vi "FilterAndReorderChannels.vi"(8 "error in (no error)":errorcluster, 10 "channels":T9[](array[typedef]), 11 "device":T1) -> (0 "error out":errorcluster, 2 "acquisition channels (in acquisition order)":T9[](array[typedef]))   [LabVIEW 2017, in "CmsAcquisition.lvlib"]
uses:
  <vilib>/addons/InsightCM/Devices/Shared/Cms/CmsAcquisition/CmsAcquisition.lvlib
  <vilib>/addons/InsightCM/MessageBus/Base/controls/R2_Channel.ctl
  <vilib>/addons/InsightCM/MessageBus/Base/controls/KeyValuePair.ctl
  <vilib>/addons/InsightCM/MessageBus/Base/controls/Metric.ctl
  <vilib>/addons/InsightCM/MessageBus/Base/controls/R2_Device.ctl
  <vilib>/addons/InsightCM/MessageBus/Base/controls/DeviceState.ctl
  <vilib>/addons/InsightCM/MessageBus/Base/controls/R2_DataGroup.ctl
  <vilib>/addons/InsightCM/MessageBus/Base/controls/OperatingState.ctl
  <vilib>/addons/InsightCM/MessageBus/Base/controls/Trigger.ctl
  <vilib>/addons/InsightCM/MessageBus/Base/controls/Condition.ctl
  <vilib>/addons/InsightCM/MessageBus/Base/controls/BurstModeTrigger.ctl
  <vilib>/addons/InsightCM/Utilities/PropertyHelpers/PropertyHelpers.lvlib
panel:
  out "hardware channel name (in acquisition order)":string[](array[string])
  out "channel IDs (in acquisition order)":string[](array[string])
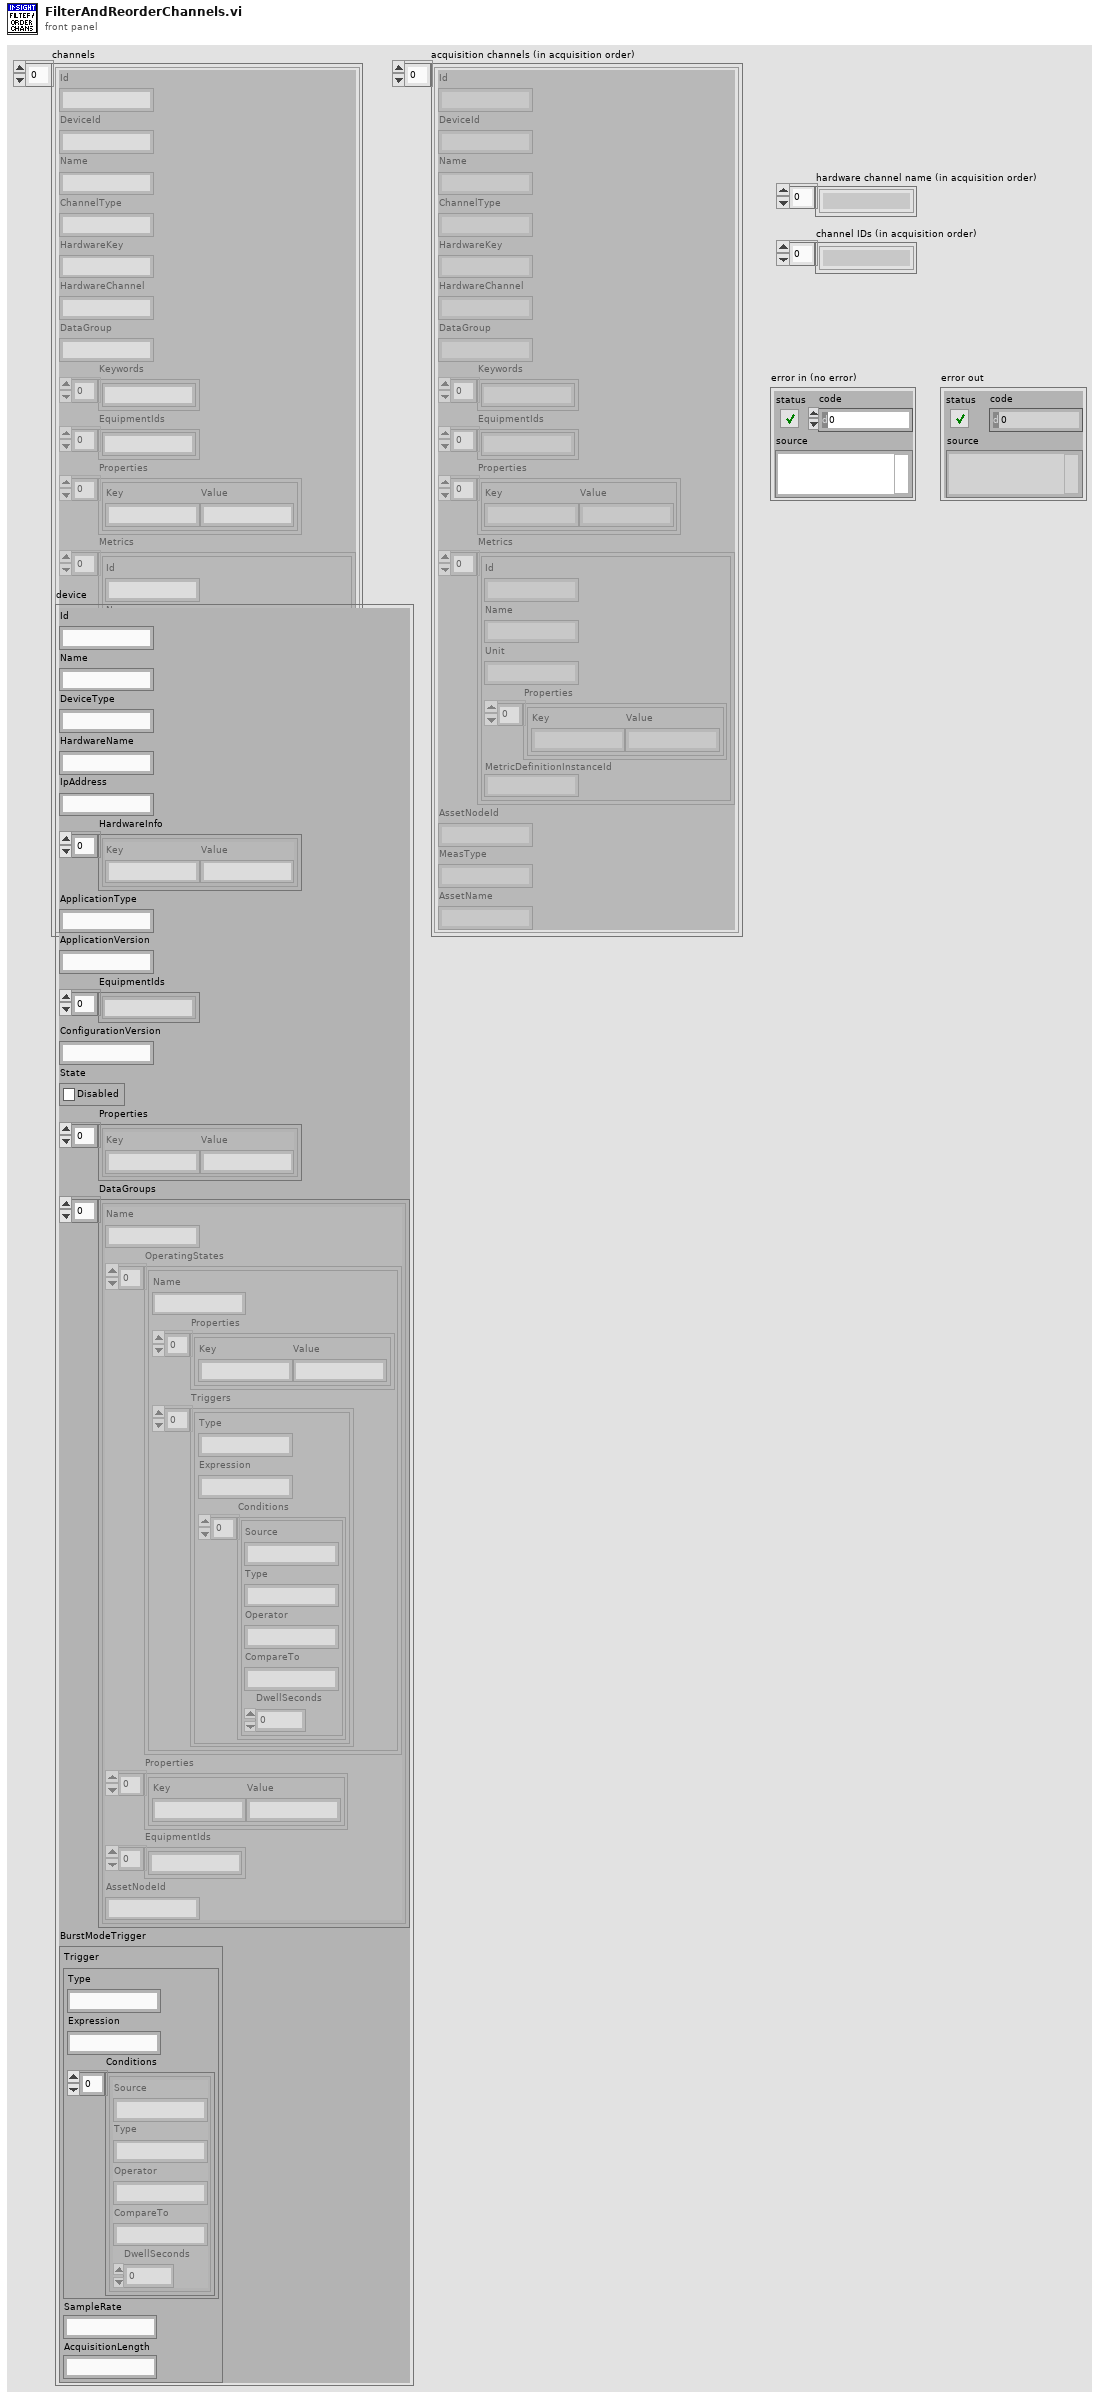
[diagram p1: front panel]
types:
  T1 = typedef "R2_Device.ctl" = cluster{"Id":string, "Name":string, "DeviceType":string, "HardwareName":string, "IpAddress":string, "HardwareInfo":T2[], "ApplicationType":string, "ApplicationVersion":string, "EquipmentIds":string[], "ConfigurationVersion":string, "State":T3, "Properties":T2[], "DataGroups":T4[], "BurstModeTrigger":T8}
  T2 = typedef "KeyValuePair.ctl" = cluster{"Key":string, "Value":string}
  T3 = typedef "DeviceState.ctl" = cluster{"Disabled":bool}
  T4 = typedef "R2_DataGroup.ctl" = cluster{"Name":string, "OperatingStates":T5[], "Properties":T2[], "EquipmentIds":string[], "AssetNodeId":string}
  T5 = typedef "OperatingState.ctl" = cluster{"Name":string, "Properties":T2[], "Triggers":T6[]}
  T6 = typedef "Trigger.ctl" = cluster{"Type":string, "Expression":string, "Conditions":T7[]}
  T7 = typedef "Condition.ctl" = cluster{"Source":string, "Type":string, "Operator":string, "CompareTo":string, "DwellSeconds":dbl}
  T8 = typedef "BurstModeTrigger.ctl" = cluster{"Trigger":T6, "SampleRate":string, "AcquisitionLength":string}
  T9 = typedef "R2_Channel.ctl" = cluster{"Id":string, "DeviceId":string, "Name":string, "ChannelType":string, "HardwareKey":string, "HardwareChannel":string, "DataGroup":string, "Keywords":string[], "EquipmentIds":string[], "Properties":T2[], "Metrics":T10[], "AssetNodeId":string, "MeasType":string, "AssetName":string}
  T10 = typedef "Metric.ctl" = cluster{"Id":string, "Name":string, "Unit":string, "Properties":T2[], "MetricDefinitionInstanceId":string}
  T11 = cluster{"HardwareChannel":string, "Id":string, "ChannelModel":T9}
  T12 = cluster{"HardwareChannel":string, "Id":string, "ChannelModel":T9}[]
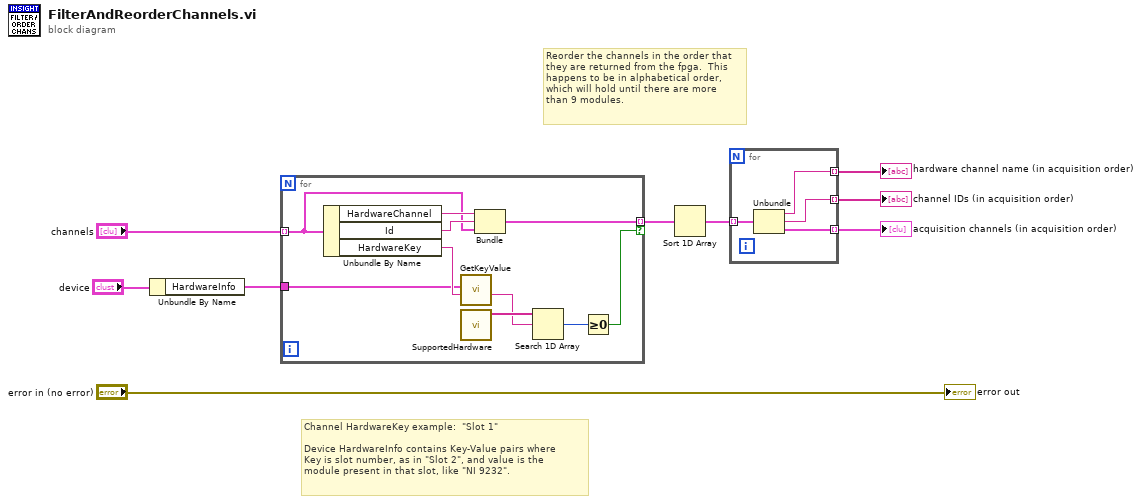
[diagram p0: block diagram]
diagram:
  # "Channel HardwareKey example:  \"Slot 1\"\n\nDevice HardwareInfo contains Key-Value pairs where\nKey is slot number, as in \"Slot 2\", and value is the\nmodule present in that slot, like \"NI 9232\"."
  # "Reorder the channels in the order that\nthey are returned from the fpga.  This\nhappens to be in alphabetical order,\nwhich will hold until there are more\nthan 9 modules."
  n1 = Unbundle By Name("device") -> ("HardwareInfo"=w1:T2[])
  n2 = for {
    tunnel: "channels" -> [w16] mode=indexing
    tunnel: [w18] -> w5 mode=indexing if=w13
    tunnel: w1 -> [w10]
    n3 = Unbundle By Name(w16) -> ("HardwareChannel"=w19:string, "Id"=w17:string, "HardwareKey"=w11:string)
    n4 = call <vilib>:"GetKeyValue.vi"("key"=w11, "key value pairs"=w10) -> ("value"=w12:string)  [unwired: 7 in, 2 out]
    n5 = call <vilib>:"SupportedHardware.vi"() -> ("Supported Hardware"=w15:string[])  [unwired: 10 in, 1 out]
    n6 = Bundle("HardwareChannel"=w19, "Id"=w17, "ChannelModel"=w16) -> (w18:T11)  [unwired: 1 in]
    n7 = Search 1D Array(1D array=w15, element=w12) -> (index of element=w14:i32)  [unwired: 1 in]
    n8 = Greater Or Equal To 0?(x=w14) -> (x >= 0?=w13:bool)
  }
  n9 = Sort 1D Array(array=w5) -> (sorted array=w6:T12)
  n10 = for {
    tunnel: w6 -> [w23] mode=indexing
    tunnel: [w22] -> w8 mode=indexing
    tunnel: [w21] -> w9 mode=indexing
    tunnel: [w20] -> w3 mode=indexing
    n11 = Unbundle(w23) -> ("HardwareChannel"=w20:string, "Id"=w22:string, "ChannelModel"=w21:T9)
  }
  "acquisition channels (in acquisition order)" <- w9
  "channel IDs (in acquisition order)" <- w8
  "hardware channel name (in acquisition order)" <- w3
  "error out" <- "error in (no error)"
